vi "Define Customized Character (5X10).vi"(8 "error in (no error)":errorcluster, 9 "customized character pattern":bool[][](array[boolean]), 10 "customized character code in":u8, 11 "HD44780 in":refnum<class "HD44780.lvclass">) -> (0 "error out":errorcluster, 2 "customized character code out":u8, 3 "HD44780 out":refnum<class "HD44780.lvclass">)   [LabVIEW 2017, in "HD44780.lvclass"]
uses:
  HD44780.lvclass
  HD44780.lvclass/HD44780.ctl
  Common/HD44780 Common.lvlib
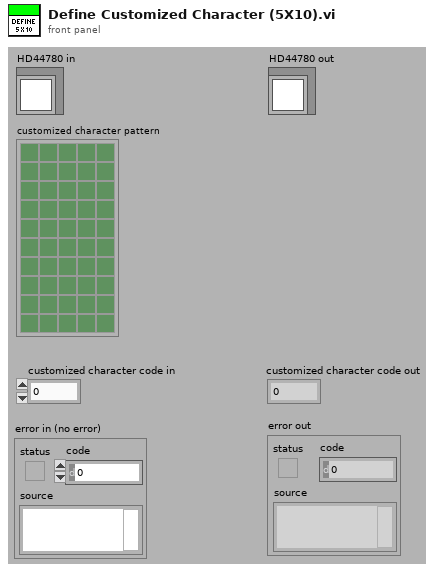
[diagram p1: front panel]
types:
  T1 = typedef "HD44780 Common.lvlib/cluster of class private data.ctl" = cluster{"FPGA VI Reference":refnum<k20>, "device index":i8, "screen size":T2, "font size":T3, "auto wrap":bool, "alignment":T4, "number of line":T5, "shift 0":i8, "entry mode 0":T6, "shift 1":i8, "entry mode 1":T6}
  T2 = typedef "HD44780 Common.lvlib/screen size.ctl" = enum8{"8x1", "8x2", "12x4", "16x1", "16x2", "16x4", "20x1", "20x2", "20x4", "24x1", "24x2", "40x2", "40x4"}
  T3 = typedef "HD44780 Common.lvlib/font size.ctl" = enum8{"5x8", "5x10"}
  T4 = typedef "HD44780 Common.lvlib/alignment.ctl" = enum16{"None", "Left", "Center", "Right"}
  T5 = typedef "HD44780 Common.lvlib/line number.ctl" = enum8{"1 line", "2 lines"}
  T6 = typedef "HD44780 Common.lvlib/entry mode.ctl" = enum8{"increment & no shift", "increment & shift", "decrement & no shift", "decrement & shift"}
  T7 = cluster{"FPGA VI Reference":refnum<k20>, "device index":i8, "screen size":enum8{"8x1", "8x2", "12x4", "16x1", "16x2", "16x4", "20x1", "20x2", "20x4", "24x1", "24x2", "40x2", "40x4"}, "font size":enum8{"5x8", "5x10"}, "auto wrap":bool, "alignment":enum16{"None", "Left", "Center", "Right"}, "number of line":enum8{"1 line", "2 lines"}, "shift 0":i8, "entry mode 0":enum8{"increment & no shift", "increment & shift", "decrement & no shift", "decrement & shift"}, "shift 1":i8, "entry mode 1":enum8{"increment & no shift", "increment & shift", "decrement & no shift", "decrement & shift"}}
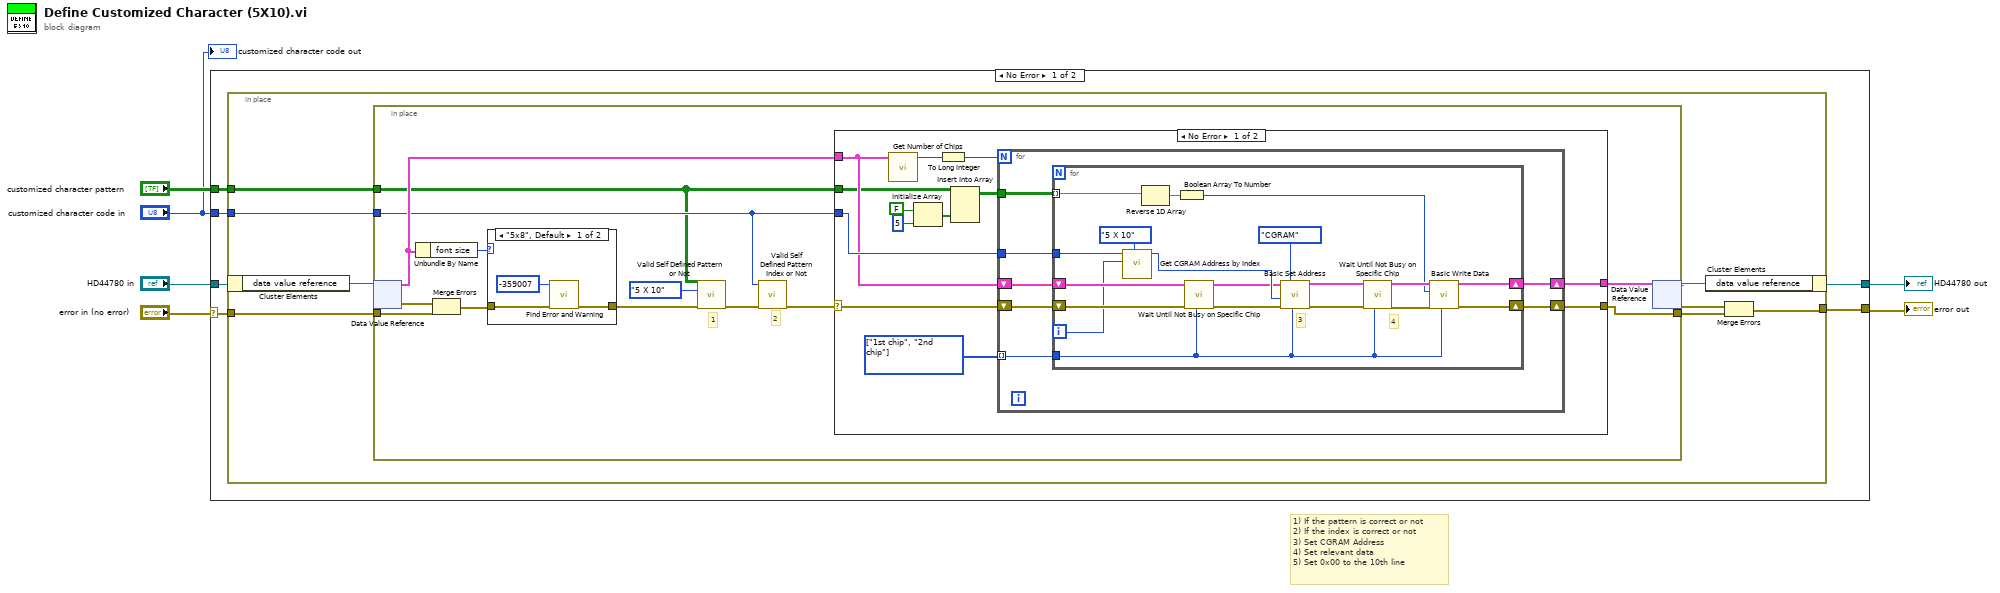
[diagram p0: block diagram]
diagram:
  # "1) If the pattern is correct or not\n2) If the index is correct or not\n3) Set CGRAM Address\n4) Set relevant data\n5) Set 0x00 to the 10th line"
  n1 = case shown="No Error" "error in (no error)" {
    selector: "error in (no error)" -> [w9 w80]
    tunnel: [w12 w80] -> w5
    tunnel: [w10 w79] -> w3
    tunnel: "HD44780 in" -> [w11 w79]
    tunnel: "customized character code in" -> [w8 _]
    tunnel: "customized character pattern" -> [w7 _]
    frame No Error {
      n2 = in-place {
        in-place-border: [w18] -> w12
        in-place-border: w9 -> [w17]
        in-place-border: w8 -> [w16]
        in-place-border: w7 -> [w15]
        n3 = in-place-cluster #1(w11) -> ("data value reference"=w20:refnum<data-value>)
        n4 = in-place {
          in-place-border: w17 -> [w26]
          in-place-border: w16 -> [w23]
          in-place-border: w15 -> [w22]
          in-place-border: [w21] -> w13
          # "2"
          # "1"
          n5 = in-place-dvr #2(w20) -> (w29:T1, w27:errorcluster)
          n6 = Unbundle By Name(w29) -> ("font size"=w24:T3)
          n7 = Merge Errors(w27, w26) -> (w25:errorcluster)
          n8 = case shown="\"5x8\", Default" w24 {
            tunnel: [w34 w37] -> w30
            tunnel: w25 -> [w35 w37]
            frame "5x8", Default {
              n9 = call "Find Error and Warning.vi"("error in (no error)"=w35, "error code"=-359007) -> ("error out"=w34:errorcluster)  [unwired: 9 in]
            }
            frame "5x10" {
            }
          }
          n10 = call "Valid Self Defined Pattern or Not.vi"("error in (no error)"=w30, "self defined pattern"=enum16{"5 X 10", "5 X 8"}."5 X 10", "customized character pattern"=w22) -> ("error out"=w33:errorcluster)  [unwired: 8 in]
          n11 = call "Valid Self Defined Pattern Index or Not.vi"("error in (no error)"=w33, "customized character code"=w23) -> ("error out"=w32:errorcluster)  [unwired: 9 in]
          n12 = case shown="No Error" w32 {
            selector: w32 -> [w49 w77]
            tunnel: w22 -> [w40 _]
            tunnel: w23 -> [w48 _]
            tunnel: w29 -> [w45 w78]
            tunnel: [w47 w78] -> w28
            tunnel: [w46 w77] -> w21
            frame No Error {
              w39 = enum16{"1st chip", "2nd chip"}[] [enum."1st chip", enum."2nd chip"] items=["1st chip", "2nd chip"]
              n13 = call "Get Number of Chips.vi"("cluster of private data in"=w45) -> ("number of chips"=w50:u8)  [unwired: 10 in]
              n14 = Initialize Array(FALSE, 5 ("dimension size")) -> (w43:bool[])
              n15 = To Long Integer(number=w50) -> (32bit integer=w44:i32)
              n16 = Insert Into Array(array=w40, new element=w43) -> (w38:bool[][])  [unwired: 2 in]
              n17 = for {
                N: w44 -> [_]
                shift-right: [w52] -> w46
                shift-left: w49 -> [w57]
                tunnel: w39 -> [w54] mode=indexing
                tunnel: w48 -> [w56]
                tunnel: w38 -> [w51]
                shift-right: [w53] -> w47
                shift-left: w45 -> [w55]
                n18 = for {
                  shift-right: [w76] -> w52
                  shift-left: w57 -> [w66]
                  tunnel: w56 -> [w70]
                  tunnel: w54 -> [w58]
                  tunnel: w51 -> [w60] mode=indexing
                  shift-right: [w74] -> w53
                  shift-left: w55 -> [w63]
                  i -> [w62]
                  # "3"
                  # "4"
                  n19 = call "Get CGRAM Address by Index.vi"("self defined pattern"=enum16{"5 X 10", "5 X 8"}."5 X 10", "index of row"=w62, "customized character index"=w70) -> ("CGRAM address"=w72:u8)  [unwired: 8 in]
                  n20 = Reverse 1D Array(array=w60) -> (reversed array=w61:bool[])
                  n21 = Boolean Array To Number(Boolean array=w61) -> (number=w59:u8)
                  n22 = call "Wait Until Not Busy on Specific Chip.vi"("chip select  (1st chip)"=w58, "error in (no error)"=w66, "cluster of private data in"=w63) -> ("error out"=w65:errorcluster, "cluster of private data out"=w64:T7)  [unwired: 7 in]
                  n23 = call "Basic Set Address.vi"("chip select  (1st chip)"=w58, "address type (DDRAM)"=enum16{"DDRAM", "CGRAM"}."CGRAM" ("address type (DD RAM)"), "error in (no error)"=w65, "address (0, 0)"=w72, "cluster of private data in"=w64) -> ("error out"=w69:errorcluster, "cluster of private data out"=w68:T7)  [unwired: 5 in]
                  n24 = call "Wait Until Not Busy on Specific Chip.vi"("chip select  (1st chip)"=w58, "error in (no error)"=w69, "cluster of private data in"=w68) -> ("error out"=w75:errorcluster, "cluster of private data out"=w67:T7)  [unwired: 7 in]
                  n25 = call "Basic Write Data.vi"("chip select  (1st chip)"=w58, "error in (no error)"=w75, "character code"=w59, "cluster of private data in"=w67) -> ("error out"=w76:errorcluster, "cluster of private data out"=w74:T7)  [unwired: 6 in]
                }
              }
            }
            frame Error {
            }
          }
          n26 = in-place-dvr #2(w28) -> (w19:refnum<data-value>, w14:errorcluster)
        }
        n27 = in-place-cluster #1("data value reference"=w19) -> (w10:refnum<class "HD44780.lvclass">)
        n28 = Merge Errors(w14, w13) -> (w18:errorcluster)
      }
    }
    frame Error {
    }
  }
  "error out" <- w5
  "HD44780 out" <- w3
  "customized character code out" <- "customized character code in"
